vi "Package Payload.vi"(11 "Destination Path":path) -> (3 "String":string)   [LabVIEW 2015]
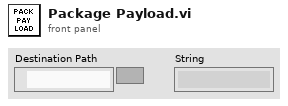
[diagram p1: front panel]
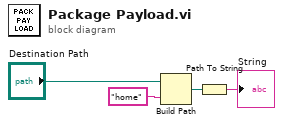
[diagram p0: block diagram]
diagram:
  n1 = Build Path(base path="Destination Path", name or relative path="home") -> (appended path=w3:path)
  n2 = Path To String(path=w3) -> (string=→"String":string)
